vi "MoveHead.vi"(8 "error in (no error)":errorcluster, 11 "Game Data in":T1) -> (0 "error out":errorcluster, 3 "Game Data out":T1)   [LabVIEW 2020]
uses:
  TypeDef/game-data.ctl
  TypeDef/tiles-key.ctl
  TypeDef/direction.ctl
  <vilib>/Utility/error.llb/Error Cluster From Error Code.vi
  <vilib>/ErrorRing/Error Ring.xnode
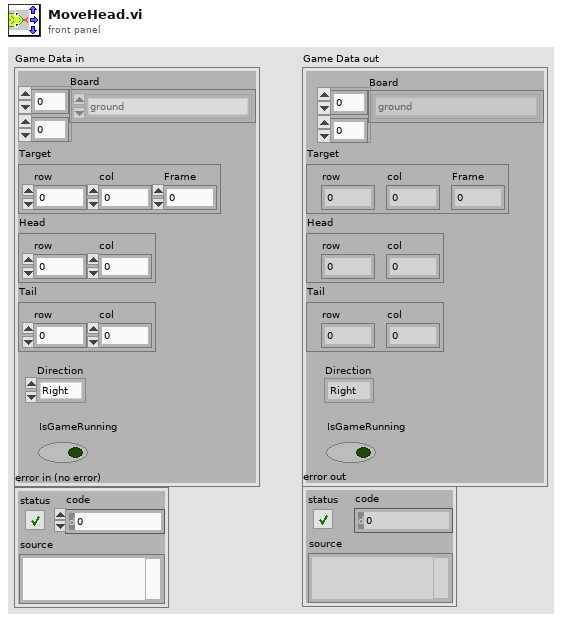
[diagram p1: front panel]
types:
  T1 = typedef "game-data.ctl" = cluster{"Board":T2[][], "Target":cluster{"row":i32, "col":i32, "Frame":i8}, "Head":cluster{"row":i32, "col":i32}, "Tail":cluster{"row":i32, "col":i32}, "Direction":T3, "IsGameRunning":bool}
  T2 = typedef "tiles-key.ctl" = enum16{"ground", "wall", "head (right)", "head (up)", "head (left)", "head (down)", "L-turn (right-up)", "L-turn (up-left)", "L-turn (left-down)", "L-turn (down-right)", "body (right)", "body (up)", "body (left)", "body (down)", "R-turn (right-down)", "R-turn (up-right)", "R-turn (left-up)", "R-turn (down-left)", "tail (right)", "tail (up)", "tail (left)", "tail (down)", "dead head (right)", "dead head (up)", "dead head (left)", "dead head (down)", "dead L-turn (right-up)", "dead L-turn (up-left)", "dead L-turn (left-down)", "dead L-turn (down-right)", "dead body (right)", "dead body (up)", "dead body (left)", "dead body (down)", "dead R-turn (right-down)", "dead R-turn (up-right)", "dead R-turn (left-up)", "dead R-turn (down-left)", "dead tail (right)", "dead tail (up)", "dead tail (left)", "dead tail (down)", "target red", "target blue", "target yellow", "target green"}
  T3 = typedef "direction.ctl" = enum16{"Right", "Up", "Left", "Down"}
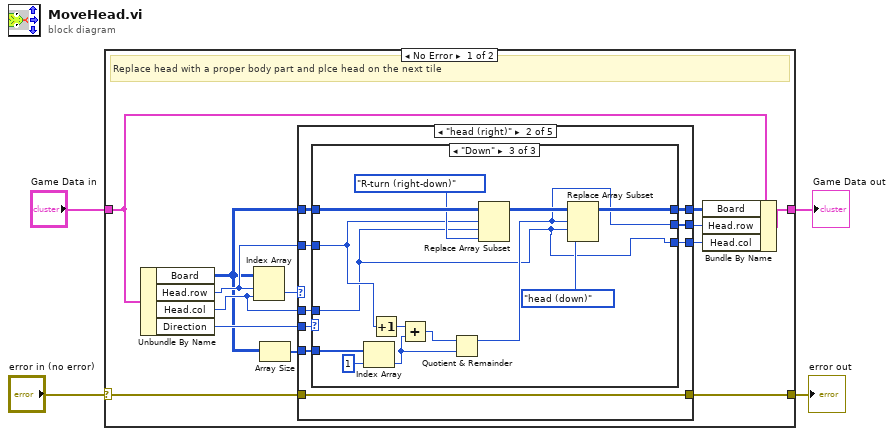
[diagram p0: block diagram]
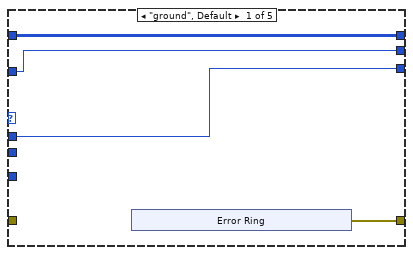
[diagram p2: hidden frame]
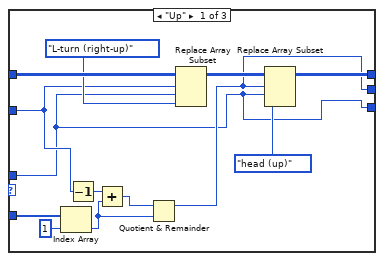
[diagram p3: hidden frame]
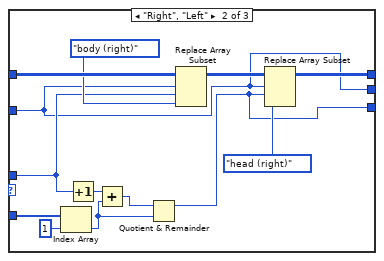
[diagram p4: hidden frame]
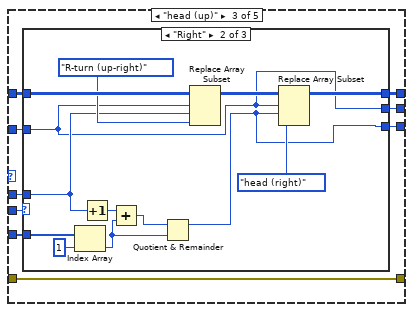
[diagram p5: hidden frame]
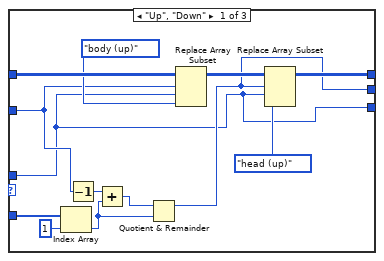
[diagram p6: hidden frame]
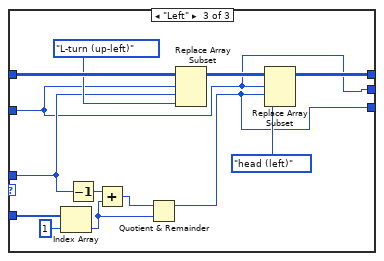
[diagram p7: hidden frame]
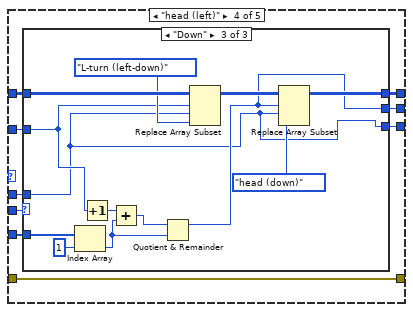
[diagram p8: hidden frame]
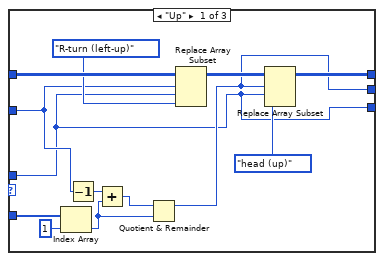
[diagram p9: hidden frame]
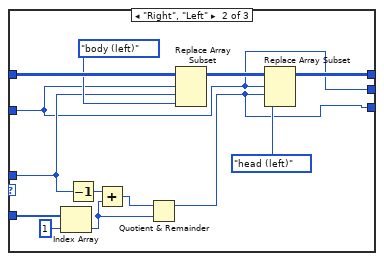
[diagram p10: hidden frame]
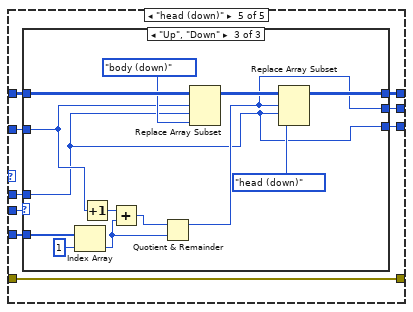
[diagram p11: hidden frame]
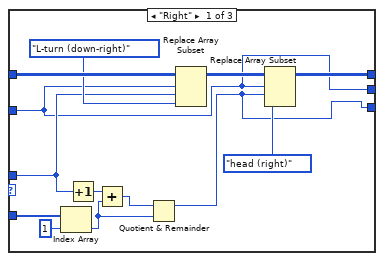
[diagram p12: hidden frame]
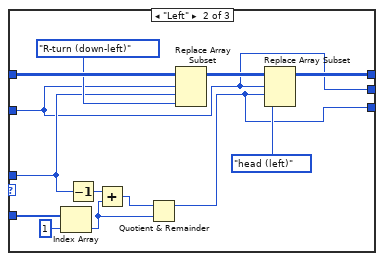
[diagram p13: hidden frame]
diagram:
  n1 = case shown="No Error" "error in (no error)" {
    selector: "error in (no error)" -> [w14 w220]
    tunnel: "Game Data in" -> [w17 w219]
    tunnel: [w16 w219] -> w3
    tunnel: [w13 w220] -> w1
    frame No Error {
      # "Replace head with a proper body part and plce head on the next tile"
      n2 = Unbundle By Name(w17) -> ("Board"=w9:T2[][], "Head.row"=w11:i32, "Head.col"=w10:i32, "Direction"=w12:T3)
      n3 = Index Array(array=w9, index (row)=w11, index (col)=w10) -> (element=w15:T2)
      n4 = Array Size(array=w9) -> (size(s)=w8:i32[])
      n5 = case shown="\"head (right)\"" w15 {
        tunnel: w14 -> [_ w35 w83 w131 w179]
        tunnel: [w21 w35 w83 w131 w179] -> w13
        tunnel: w12 -> [_ w34 w82 w130 w178]
        tunnel: w9 -> [w20 w31 w79 w127 w175]
        tunnel: w11 -> [w19 w33 w81 w129 w177]
        tunnel: w10 -> [w18 w32 w80 w128 w176]
        tunnel: w8 -> [_ w30 w78 w126 w174]
        tunnel: [w20 w29 w77 w125 w173] -> w7
        tunnel: [w19 w28 w76 w124 w172] -> w6
        tunnel: [w18 w27 w75 w123 w171] -> w5
        frame "ground", Default {
          n6 = xnode "Error Ring"() -> ("error out"=w21:errorcluster)
        }
        frame "head (right)" {
          n7 = case shown="\"Down\"" w34 {
            tunnel: w33 -> [w43 w50 w69]
            tunnel: w32 -> [w36 w51 w62]
            tunnel: w31 -> [w46 w59 w72]
            tunnel: w30 -> [w48 w61 w74]
            tunnel: [w38 w52 w64] -> w29
            tunnel: [w37 w50 w63] -> w28
            tunnel: [w36 w49 w62] -> w27
            frame "Up" {
              n8 = Index Array(array=w48, index=1) -> (element=w42:i32)
              n9 = Decrement(x=w43) -> (x-1=w41:i32)
              n10 = Add(x=w41, y=w42) -> (x+y=w44:i32)
              n11 = Quotient & Remainder(x=w44, y=w42) -> (x-y*floor(x/y)=w37:i32)  [unwired: 1 out]
              n12 = Replace Array Subset(array=w46, new element=tiles-key."L-turn (right-up)" ("new element/subarray"), index (row)=w43, index (col)=w36) -> (w40:T2[][])
              n13 = Replace Array Subset(array=w40, new element=tiles-key."head (up)" ("new element/subarray"), index (row)=w37, index (col)=w36) -> (w38:T2[][])
            }
            frame "Right", "Left" {
              n14 = Index Array(array=w61, index=1) -> (element=w56:i32)
              n15 = Increment(x=w51) -> (x+1=w55:i32)
              n16 = Add(x=w55, y=w56) -> (x+y=w57:i32)
              n17 = Quotient & Remainder(x=w57, y=w56) -> (x-y*floor(x/y)=w49:i32)  [unwired: 1 out]
              n18 = Replace Array Subset(array=w59, new element=tiles-key."body (right)" ("new element/subarray"), index (row)=w50, index (col)=w51) -> (w54:T2[][])
              n19 = Replace Array Subset(array=w54, new element=tiles-key."head (right)" ("new element/subarray"), index (row)=w50, index (col)=w49) -> (w52:T2[][])
            }
            frame "Down" {
              n20 = Index Array(array=w74, index=1) -> (element=w68:i32)
              n21 = Increment(x=w69) -> (x+1=w67:i32)
              n22 = Add(x=w67, y=w68) -> (x+y=w70:i32)
              n23 = Quotient & Remainder(x=w70, y=w68) -> (x-y*floor(x/y)=w63:i32)  [unwired: 1 out]
              n24 = Replace Array Subset(array=w72, new element=tiles-key."R-turn (right-down)" ("new element/subarray"), index (row)=w69, index (col)=w62) -> (w66:T2[][])
              n25 = Replace Array Subset(array=w66, new element=tiles-key."head (down)" ("new element/subarray"), index (row)=w63, index (col)=w62) -> (w64:T2[][])
            }
          }
        }
        frame "head (up)" {
          n26 = case shown="\"Right\"" w82 {
            tunnel: w81 -> [w91 w98 w111]
            tunnel: w80 -> [w84 w99 w112]
            tunnel: w79 -> [w94 w107 w120]
            tunnel: w78 -> [w96 w109 w122]
            tunnel: [w86 w100 w113] -> w77
            tunnel: [w85 w98 w111] -> w76
            tunnel: [w84 w97 w110] -> w75
            frame "Up", "Down" {
              n27 = Index Array(array=w96, index=1) -> (element=w90:i32)
              n28 = Decrement(x=w91) -> (x-1=w89:i32)
              n29 = Add(x=w89, y=w90) -> (x+y=w92:i32)
              n30 = Quotient & Remainder(x=w92, y=w90) -> (x-y*floor(x/y)=w85:i32)  [unwired: 1 out]
              n31 = Replace Array Subset(array=w94, new element=tiles-key."body (up)" ("new element/subarray"), index (row)=w91, index (col)=w84) -> (w88:T2[][])
              n32 = Replace Array Subset(array=w88, new element=tiles-key."head (up)" ("new element/subarray"), index (row)=w85, index (col)=w84) -> (w86:T2[][])
            }
            frame "Right" {
              n33 = Index Array(array=w109, index=1) -> (element=w104:i32)
              n34 = Increment(x=w99) -> (x+1=w103:i32)
              n35 = Add(x=w103, y=w104) -> (x+y=w105:i32)
              n36 = Quotient & Remainder(x=w105, y=w104) -> (x-y*floor(x/y)=w97:i32)  [unwired: 1 out]
              n37 = Replace Array Subset(array=w107, new element=tiles-key."R-turn (up-right)" ("new element/subarray"), index (row)=w98, index (col)=w99) -> (w102:T2[][])
              n38 = Replace Array Subset(array=w102, new element=tiles-key."head (right)" ("new element/subarray"), index (row)=w98, index (col)=w97) -> (w100:T2[][])
            }
            frame "Left" {
              n39 = Index Array(array=w122, index=1) -> (element=w117:i32)
              n40 = Decrement(x=w112) -> (x-1=w116:i32)
              n41 = Add(x=w116, y=w117) -> (x+y=w118:i32)
              n42 = Quotient & Remainder(x=w118, y=w117) -> (x-y*floor(x/y)=w110:i32)  [unwired: 1 out]
              n43 = Replace Array Subset(array=w120, new element=tiles-key."L-turn (up-left)" ("new element/subarray"), index (row)=w111, index (col)=w112) -> (w115:T2[][])
              n44 = Replace Array Subset(array=w115, new element=tiles-key."head (left)" ("new element/subarray"), index (row)=w111, index (col)=w110) -> (w113:T2[][])
            }
          }
        }
        frame "head (left)" {
          n45 = case shown="\"Down\"" w130 {
            tunnel: w129 -> [w139 w146 w165]
            tunnel: w128 -> [w132 w147 w158]
            tunnel: w127 -> [w142 w155 w168]
            tunnel: w126 -> [w144 w157 w170]
            tunnel: [w134 w148 w160] -> w125
            tunnel: [w133 w146 w159] -> w124
            tunnel: [w132 w145 w158] -> w123
            frame "Up" {
              n46 = Index Array(array=w144, index=1) -> (element=w138:i32)
              n47 = Decrement(x=w139) -> (x-1=w137:i32)
              n48 = Add(x=w137, y=w138) -> (x+y=w140:i32)
              n49 = Quotient & Remainder(x=w140, y=w138) -> (x-y*floor(x/y)=w133:i32)  [unwired: 1 out]
              n50 = Replace Array Subset(array=w142, new element=tiles-key."R-turn (left-up)" ("new element/subarray"), index (row)=w139, index (col)=w132) -> (w136:T2[][])
              n51 = Replace Array Subset(array=w136, new element=tiles-key."head (up)" ("new element/subarray"), index (row)=w133, index (col)=w132) -> (w134:T2[][])
            }
            frame "Right", "Left" {
              n52 = Index Array(array=w157, index=1) -> (element=w152:i32)
              n53 = Decrement(x=w147) -> (x-1=w151:i32)
              n54 = Add(x=w151, y=w152) -> (x+y=w153:i32)
              n55 = Quotient & Remainder(x=w153, y=w152) -> (x-y*floor(x/y)=w145:i32)  [unwired: 1 out]
              n56 = Replace Array Subset(array=w155, new element=tiles-key."body (left)" ("new element/subarray"), index (row)=w146, index (col)=w147) -> (w150:T2[][])
              n57 = Replace Array Subset(array=w150, new element=tiles-key."head (left)" ("new element/subarray"), index (row)=w146, index (col)=w145) -> (w148:T2[][])
            }
            frame "Down" {
              n58 = Index Array(array=w170, index=1) -> (element=w164:i32)
              n59 = Increment(x=w165) -> (x+1=w163:i32)
              n60 = Add(x=w163, y=w164) -> (x+y=w166:i32)
              n61 = Quotient & Remainder(x=w166, y=w164) -> (x-y*floor(x/y)=w159:i32)  [unwired: 1 out]
              n62 = Replace Array Subset(array=w168, new element=tiles-key."L-turn (left-down)" ("new element/subarray"), index (row)=w165, index (col)=w158) -> (w162:T2[][])
              n63 = Replace Array Subset(array=w162, new element=tiles-key."head (down)" ("new element/subarray"), index (row)=w159, index (col)=w158) -> (w160:T2[][])
            }
          }
        }
        frame "head (down)" {
          n64 = case shown="\"Up\", \"Down\"" w178 {
            tunnel: w177 -> [w181 w194 w213]
            tunnel: w176 -> [w182 w195 w206]
            tunnel: w175 -> [w190 w203 w216]
            tunnel: w174 -> [w192 w205 w218]
            tunnel: [w183 w196 w208] -> w173
            tunnel: [w181 w194 w207] -> w172
            tunnel: [w180 w193 w206] -> w171
            frame "Right" {
              n65 = Index Array(array=w192, index=1) -> (element=w187:i32)
              n66 = Increment(x=w182) -> (x+1=w186:i32)
              n67 = Add(x=w186, y=w187) -> (x+y=w188:i32)
              n68 = Quotient & Remainder(x=w188, y=w187) -> (x-y*floor(x/y)=w180:i32)  [unwired: 1 out]
              n69 = Replace Array Subset(array=w190, new element=tiles-key."L-turn (down-right)" ("new element/subarray"), index (row)=w181, index (col)=w182) -> (w185:T2[][])
              n70 = Replace Array Subset(array=w185, new element=tiles-key."head (right)" ("new element/subarray"), index (row)=w181, index (col)=w180) -> (w183:T2[][])
            }
            frame "Left" {
              n71 = Index Array(array=w205, index=1) -> (element=w200:i32)
              n72 = Decrement(x=w195) -> (x-1=w199:i32)
              n73 = Add(x=w199, y=w200) -> (x+y=w201:i32)
              n74 = Quotient & Remainder(x=w201, y=w200) -> (x-y*floor(x/y)=w193:i32)  [unwired: 1 out]
              n75 = Replace Array Subset(array=w203, new element=tiles-key."R-turn (down-left)" ("new element/subarray"), index (row)=w194, index (col)=w195) -> (w198:T2[][])
              n76 = Replace Array Subset(array=w198, new element=tiles-key."head (left)" ("new element/subarray"), index (row)=w194, index (col)=w193) -> (w196:T2[][])
            }
            frame "Up", "Down" {
              n77 = Index Array(array=w218, index=1) -> (element=w212:i32)
              n78 = Increment(x=w213) -> (x+1=w211:i32)
              n79 = Add(x=w211, y=w212) -> (x+y=w214:i32)
              n80 = Quotient & Remainder(x=w214, y=w212) -> (x-y*floor(x/y)=w207:i32)  [unwired: 1 out]
              n81 = Replace Array Subset(array=w216, new element=tiles-key."body (down)" ("new element/subarray"), index (row)=w213, index (col)=w206) -> (w210:T2[][])
              n82 = Replace Array Subset(array=w210, new element=tiles-key."head (down)" ("new element/subarray"), index (row)=w207, index (col)=w206) -> (w208:T2[][])
            }
          }
        }
      }
      n83 = Bundle By Name(cluster=w17, "Board"=w7, "Head.row"=w6, "Head.col"=w5) -> (w16:T1)
    }
    frame Error {
    }
  }
  "Game Data out" <- w3
  "error out" <- w1
